vi "SVT Exp Avg Level (1 Ch).vi"(6 "restart averaging (F)":bool, 8 "error in (no error)":errorcluster, 9 "time constant [ms]":dbl=125.0 format="%.2f", 10 "exponential mode":enum16{"Slow", "Fast", "Impulse", "Custom"}(ring)=enum."Fast", 11 "scaled signal [EU]":waveform(dbl)) -> (0 "error out":errorcluster, 1 "actual time constant [ms]":dbl=nan format="%.2f", 2 "unit label":string, 3 "exp avg level [EU rms]":waveform(dbl))   [LabVIEW 2017]
doc: "Computes the exponential average level of <B>scaled signal [EU]</B> or <B>even angle signal [EU]</B>. You can use this polymorphic VI to compute the exponential average level for a single channel or for N channels, or for a single channel or N channels of angular resampled data. The data type you wire to the <B>scaled signal [EU]</B> or <B>even angle signal [EU]</B> input determines the polymorphic instance to use."
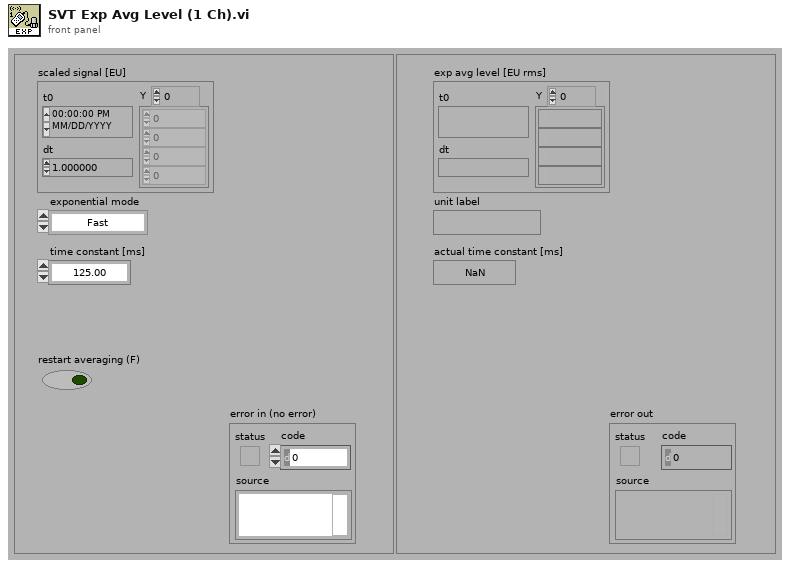
[diagram p1: front panel]
types:
  T1 = enum16{"RMS", "Running RMS", "Exp avg  ", "Dec exp avg ", "Peak", "Crest"}
  T2 = enum16{"Reset filter", "Restart averaging", "Continue processing"}
  T3 = typedef "svc_Channel Info.ctl" = cluster{"sensor sensitivity":dbl, "engineering units":T4, "dB reference":dbl, "custom label":string, "weighting filter":T5, "pregain":dbl}
  T4 = typedef "svc_Engineering Units Text Ring.ctl" = u16
  T5 = typedef "svc_Weighting Filter Text Ring.ctl" = u16
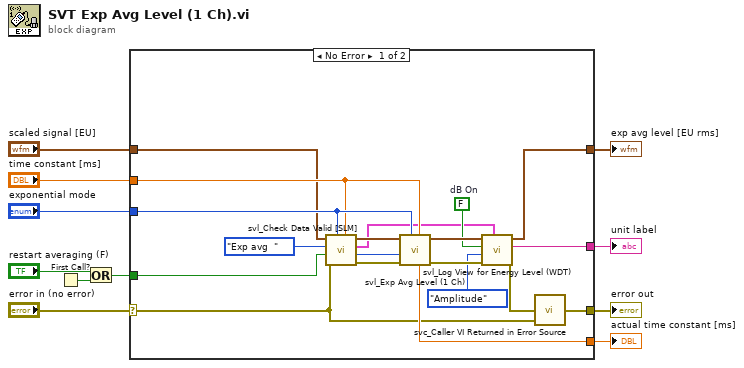
[diagram p0: block diagram]
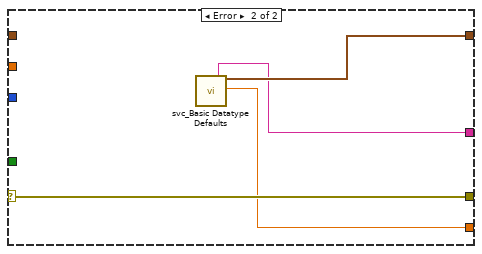
[diagram p2: hidden frame]
diagram:
  n1 = First Call?() -> (First Call?: T/F=w6:bool)
  n2 = Or(x="restart averaging (F)", y=w6) -> (x .or. y?=w5:bool)
  n3 = case shown="No Error" "error in (no error)" {
    selector: "error in (no error)" -> [w12 w34]
    tunnel: [w19 w34] -> w11
    tunnel: [w29 w31] -> w10
    tunnel: [w14 w33] -> w9
    tunnel: "scaled signal [EU]" -> [w13 _]
    tunnel: w5 -> [w18 _]
    tunnel: "exponential mode" -> [w22 _]
    tunnel: "time constant [ms]" -> [w21 _]
    tunnel: [w20 w32] -> w2
    frame No Error {
      w26 = FALSE  # dB On
      n4 = call <vilib>:"svl_Check Data Valid [SLM].vi"("time constant [ms]"=w21, "exponential mode"=w22, "error in (no error)"=w12, "restart averaging (F)"=w18, "Level Analysis"=T1."Exp avg  ", "scaled signal [EU]"=w13) -> ("error out"=w25:errorcluster, "processing state"=w23:T2, "channel info"=w15:T3, "dup scaled signal [EU]"=w16:waveform(dbl))  [unwired: 2 in]
      n5 = call <vilib>:"svl_Exp Avg Level (1 Ch).vi"("timeConstant"=w21, "exponential mode"=w22, "error in (no error)"=w25, "processing state"=w23, "scaledSignal"=w16) -> ("error out"=w28:errorcluster, "scaledSignal"=w27:waveform(dbl), "actual time constant [ms]"=w20:dbl)  [unwired: 3 in, 1 out]
      n6 = call <vilib>:"svl_Log View for Energy Level (WDT).vi"("channel info"=w15, "error in (no error)"=w28, "view mode"=enum16{"Power", "Amplitude"}."Amplitude", "dB On (T)"=w26, "scaledSignal"=w27) -> ("error out"=w30:errorcluster, "unit label"=w29:string, "scaledSignal"=w14:waveform(dbl))  [unwired: 4 in]
      n7 = call <vilib>:"svc_Caller VI Returned in Error Source.vi"("warning input to caller"=w12, "error in (no error)"=w30) -> ("error out"=w19:errorcluster)  [unwired: 3 in]
    }
    frame Error {
      n8 = call <vilib>:"svc_Basic Datatype Defaults.vi"() -> ("empty string"=w31:string, "empty waveform"=w33:waveform(dbl), "NaN"=w32:dbl)  [unwired: 7 in, 10 out]
    }
  }
  "exp avg level [EU rms]" <- w9
  "actual time constant [ms]" <- w2
  "unit label" <- w10
  "error out" <- w11
